vi "reql_db_drop.vi"(6 "ms timeout (0:default)":i32, 7 "db name":string, 8 "error in (no error)":errorcluster, 11 "rethinkdb in":refnum<class "RethinkDB.lvclass">) -> (0 "error out":errorcluster, 2 "db exists?":bool, 3 "rethinkdb out":refnum<class "RethinkDB.lvclass">, 4 "response":variant)   [LabVIEW 2017, in "rethinkdb.lvlib"]
uses:
  rethinkdb.lvlib
  RethinkDB.lvclass
  ql2_query.ctl
  ql2_term.ctl
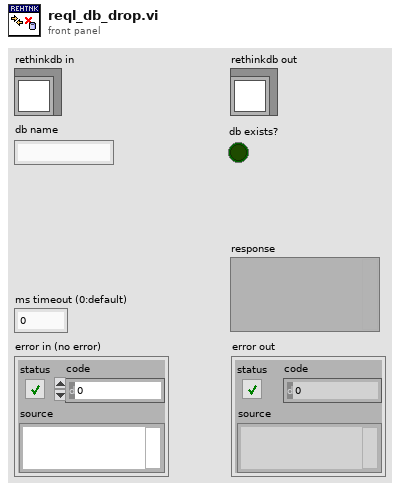
[diagram p1: front panel]
types:
  T1 = typedef "rethinkdb.lvlib/ql2_term.ctl" = enum8{"ADD", "AND", "APPEND", "APRIL", "ARGS", "ASC", "AUGUST", "AVG", "BETWEEN", "BETWEEN_DEPRECATED", "BINARY", "BIT_AND", "BIT_NOT", "BIT_OR", "BIT_SAL", "BIT_SAR", "BIT_XOR", "BRACKET", "BRANCH", "CEIL", "CHANGES", "CHANGE_AT", "CIRCLE", "COERCE_TO", "CONCAT_MAP", "CONFIG", "CONTAINS", "COUNT", "DATE", "DATUM", "DAY", "DAY_OF_WEEK", "DAY_OF_YEAR", "DB", "DB_CREATE", "DB_DROP", "DB_LIST", "DECEMBER", "DEFAULT", "DELETE", "DELETE_AT", "DESC", "DIFFERENCE", "DISTANCE", "DISTINCT", "DIV", "DOWNCASE", "DURING", "EPOCH_TIME", "EQ", "EQ_JOIN", "ERROR", "FEBRUARY", "FILL", "FILTER", "FLOOR", "FOLD", "FOR_EACH", "FRIDAY", "FUNC", "FUNCALL", "GE", "GEOJSON", "GET", "GET_ALL", "GET_FIELD", "GET_INTERSECTING", "GET_NEAREST", "GET_WRITE_HOOK", "GRANT", "GROUP", "GT", "HAS_FIELDS", "HOURS", "HTTP", "IMPLICIT_VAR", "INCLUDES", "INDEX_CREATE", "INDEX_DROP", "INDEX_LIST", "INDEX_RENAME", "INDEX_STATUS", "INDEX_WAIT", "INFO", "INNER_JOIN", "INSERT", "INSERT_AT", "INTERSECTS", "IN_TIMEZONE", "ISO8601", "IS_EMPTY", "JANUARY", "JAVASCRIPT", "JSON", "JULY", "JUNE", "KEYS", "LE", "LIMIT", "LINE", "LITERAL", "LT", "MAKE_ARRAY", "MAKE_OBJ", "MAP", "MARCH", "MATCH", "MAX", "MAXVAL", "MAY", "MERGE", "MIN", "MINUTES", "MINVAL", "MOD", "MONDAY", "MONTH", "MUL", "NE", "NOT", "NOVEMBER", "NOW", "NTH", "OBJECT", "OCTOBER", "OFFSETS_OF", "OR", "ORDER_BY", "OUTER_JOIN", "PLUCK", "POINT", "POLYGON", "POLYGON_SUB", "PREPEND", "RANDOM", "RANGE", "REBALANCE", "RECONFIGURE", "REDUCE", "REPLACE", "ROUND", "SAMPLE", "SATURDAY", "SECONDS", "SEPTEMBER", "SET_DIFFERENCE", "SET_INSERT", "SET_INTERSECTION", "SET_UNION", "SET_WRITE_HOOK", "SKIP", "SLICE", "SPLICE_AT", "SPLIT", "STATUS", "SUB", "SUM", "SUNDAY", "SYNC", "TABLE", "TABLE_CREATE", "TABLE_DROP", "TABLE_LIST", "THURSDAY", "TIME", "TIMEZONE", "TIME_OF_DAY", "TO_EPOCH_TIME", "TO_GEOJSON", "TO_ISO8601", "TO_JSON_STRING", "TUESDAY", "TYPE_OF", "UNGROUP", "UNION", "UPCASE", "UPDATE", "UUID", "VALUES", "VAR", "WAIT", "WEDNESDAY", "WITHOUT", "WITH_FIELDS", "YEAR", "ZIP", "invalid"}
  T2 = typedef "rethinkdb.lvlib/ql2_query.ctl" = enum8{"START", "CONTINUE", "STOP", "NOREPLY_WAIT", "SERVER_INFO", "invalid"}
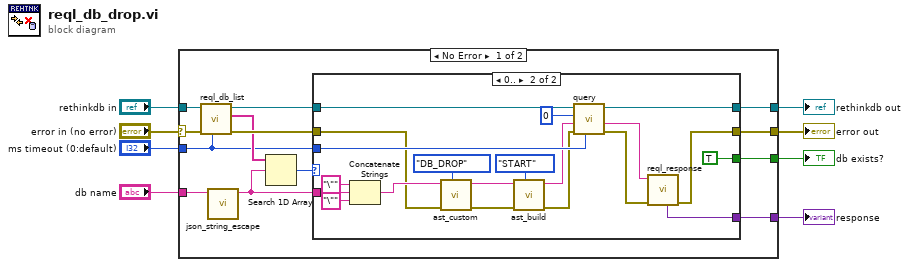
[diagram p0: block diagram]
diagram:
  n1 = case shown="No Error" "error in (no error)" {
    selector: "error in (no error)" -> [w18 w45]
    tunnel: "rethinkdb in" -> [w16 w44]
    tunnel: [w21 w44] -> w6
    tunnel: "ms timeout (0:default)" -> [w9 _]
    tunnel: [w19 w45] -> w4
    tunnel: "db name" -> [w20 _]
    tunnel: [w11 _] -> w2
    tunnel: [w10 _] -> w1
    frame No Error {
      n2 = call "reql_db_list.vi"("ms timeout (0:default)"=w9, "error in (no error)"=w18, "rethinkdb in"=w16) -> ("error out"=w17:errorcluster, "db list"=w14:string[], "rethinkdb out"=w15:refnum<class "RethinkDB.lvclass">)  [unwired: 5 in, 1 out]
      n3 = call "json_string_escape.vi"("string"=w20) -> ("escaped string"=w13:string)  [unwired: 10 in]
      n4 = Search 1D Array(1D array=w14, element=w13) -> (index of element=w12:i32)  [unwired: 1 in]
      n5 = case shown="0.." w12 {
        tunnel: [w23 w43] -> w21
        tunnel: w9 -> [_ w42]
        tunnel: [w22 w36] -> w19
        tunnel: w17 -> [w22 w24]
        tunnel: w15 -> [w23 w35]
        tunnel: w13 -> [_ w34]
        tunnel: [_ TRUE] -> w11
        tunnel: [_ w32] -> w10
        frame ..-1 {
        }
        frame 0.. {
          n6 = Concatenate Strings("\"" ("string"), w34, "\"" ("string")) -> (w25:string)
          n7 = call "ast_custom.vi"("term_type"=ql2_term."DB_DROP", "error in (no error)"=w24, "arg0"=w25) -> ("error out"=w27:errorcluster, "r"=w26:string)  [unwired: 7 in]
          n8 = call "ast_build.vi"("query_type (START)"=ql2_query."START" ("query_type"), "error in (no error)"=w27, "term"=w26) -> ("error out"=w30:errorcluster, "query"=w29:string)  [unwired: 7 in]
          n9 = call "query.vi"("ms timeout (0:default)"=w42, "error in (no error)"=w30, "query"=w29, "token in (random)"=u64 0, "rethinkdb in"=w35) -> ("error out"=w40:errorcluster, "response"=w39:string, "rethinkdb out"=w43:refnum<class "RethinkDB.lvclass">)  [unwired: 3 in, 1 out]
          n10 = call "reql_response.vi"("error in (no error)"=w40, "response"=w39) -> ("error out"=w36:errorcluster, "response"=w32:variant)  [unwired: 7 in, 1 out]
        }
      }
    }
    frame Error {
    }
  }
  "error out" <- w4
  "rethinkdb out" <- w6
  "db exists?" <- w2
  "response" <- w1
